vi "proxy_for_client_plugin.vi"(8 "error in":errorcluster, 11 "config":string) -> (0 "No error":errorcluster)   [LabVIEW 2026]
doc: "Demonstrates the use of the OS IP Stack TCP functions to connect to a TCP server VI and receive data, via a proxy server running within the XNET IP Stack."
panel:
  in  "file path (use dialog)":path=path "C:/DEV/emea-tra-iPerf_bus_load_test/support/iperf_proxies/iperf_proxies/iperf_client.json"
  in  "stop":bool
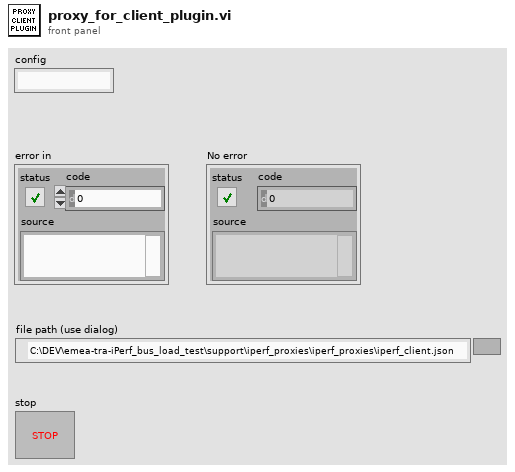
[diagram p1: front panel]
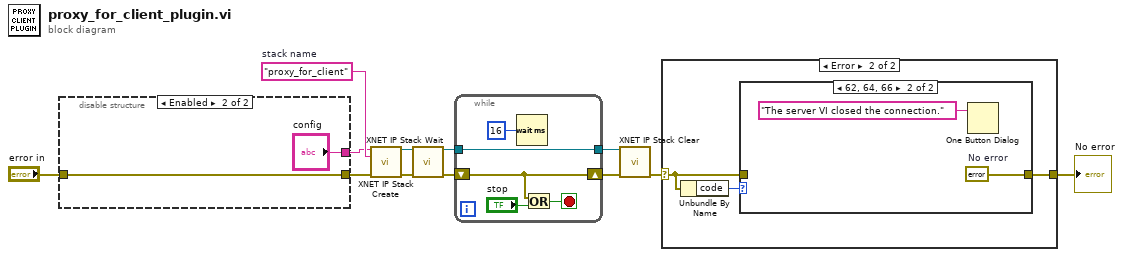
[diagram p0: block diagram]
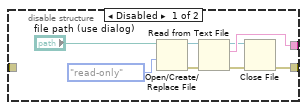
[diagram p2: hidden frame]
diagram:
  w9 = "proxy_for_client"  # stack name
  n1 = disable-structure shown="Enabled" {
    disable-tunnel: [w16 "config"] -> w4
    disable-tunnel: [w13 w21] -> w3
    disable-tunnel: "error in" -> [_ w21]
    frame Disabled {
      n2 = Open/Create/Replace File(file path (use dialog)="file path (use dialog)", access (0:read/write)=enum16{"read/write", "read-only", "write-only"}."read-only") -> (refnum out=w18:refnum<file>, error out=w17:errorcluster)  [unwired: 4 in, 1 out]
      n3 = Read from Text File(file (use dialog)=w18, error in=w17) -> (refnum out=w15:refnum<file>, text=w16:string, error out=w14:errorcluster)  [unwired: 2 in, 1 out]
      n4 = Close File(refnum=w15, error in=w14) -> (error out=w13:errorcluster)  [unwired: 1 out]
    }
    frame Enabled {
    }
  }
  n5 = call <vilib>:"XNET IP Stack Create.vi"("config"=w4, "stack name"=w9, "error in"=w3) -> ("stack out"=w11:refnum<k21>, "error out"=w12:errorcluster)  [unwired: 11 in]
  n6 = call <vilib>:"XNET IP Stack Wait.vi"("stack in"=w11, "error in"=w12) -> ("stack out"=w6:refnum<k21>, "error out"=w7:errorcluster)  [unwired: 12 in]
  n7 = while {
    shift-right: [w27] -> w8
    shift-left: w7 -> [w27]
    tunnel: w6 -> [w24]
    tunnel: [w24] -> w5
    stop <- w25 stop-if-true
    n8 = Wait (ms)(milliseconds to wait=u32 16) -> ()  [unwired: 1 out]
    n9 = Or(x=w27, y="stop") -> (x .or. y?=w25:bool)
  }
  n10 = call <vilib>:"XNET IP Stack Clear.vi"("stack"=w5, "error in"=w8) -> ("error out"=w10:errorcluster)  [unwired: 13 in]
  n11 = case shown="Error" w10 {
    selector: w10 -> [w28 w30]
    tunnel: [w28 w29] -> w1
    frame No Error {
    }
    frame Error {
      n12 = Unbundle By Name(w30) -> ("code"=w31:i32)
      n13 = case shown="62, 64, 66" w31 {
        tunnel: w30 -> [w32 _]
        tunnel: [w32 w34] -> w29
        frame Default {
        }
        frame 62, 64, 66 {
          w34 = errorcluster {"status"=FALSE, "code"=0, "source"=""}  # No error
          n14 = One Button Dialog(message="The server VI closed the connection." ("Server Closed")) -> ()  [unwired: 1 in, 1 out]
        }
      }
    }
  }
  "No error" <- w1
